vi "Merge 2 lines in array.vi"(8 "Index of 2nd line to merge":i32, 9 "Index of 1st line to merge":i32, 11 "Lines":T1[](array[typedef])) -> (3 "Merged Lines":T1[](array[typedef]))   [LabVIEW 2017]
uses:
  Vector Library/Line.ctl
  Vector Library/Vector.ctl
panel:
  out "Line to Merge":cluster{"Points":cluster{"X":dbl, "Y":dbl}[]}
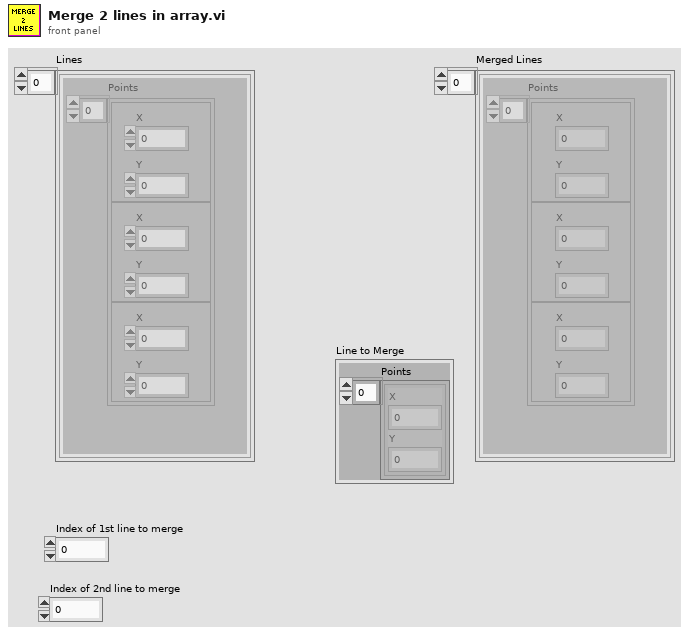
[diagram p1: front panel]
types:
  T1 = typedef "Line.ctl" = cluster{"Points":T2[]}
  T2 = typedef "Vector.ctl" = cluster{"X":dbl, "Y":dbl}
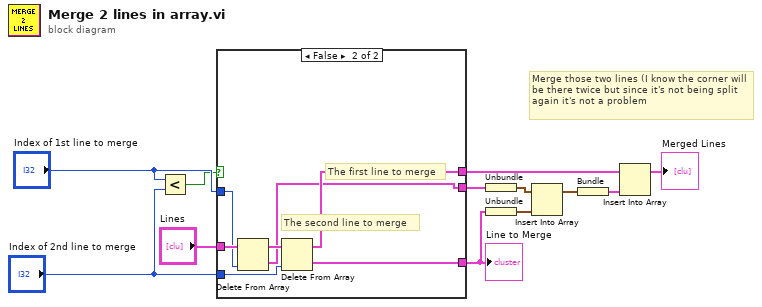
[diagram p0: block diagram]
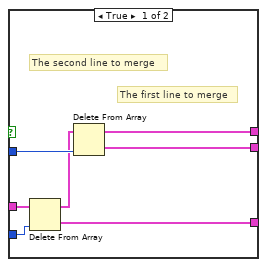
[diagram p2: hidden frame]
diagram:
  # "Merge those two lines (I know the corner will be there twice but since it's not being split again it's not a problem"
  n1 = Less?(x="Index of 1st line to merge", y="Index of 2nd line to merge") -> (x < y?=w4:bool)
  n2 = case shown="False" w4 {
    tunnel: "Lines" -> [w19 w23]
    tunnel: [w14 w20] -> w11
    tunnel: [w18 w26] -> w9
    tunnel: [w13 w25] -> w3
    tunnel: "Index of 1st line to merge" -> [w16 w22]
    tunnel: "Index of 2nd line to merge" -> [w17 w24]
    frame True {
      # "The first line to merge"
      # "The second line to merge"
      n3 = Delete From Array(array=w19, index=w17) -> (deleted portion=w18:T1, array with subset deleted=w15:T1[])  [unwired: 1 in]
      n4 = Delete From Array(array=w15, index=w16) -> (deleted portion=w14:T1, array with subset deleted=w13:T1[])  [unwired: 1 in]
    }
    frame False {
      # "The first line to merge"
      # "The second line to merge"
      n5 = Delete From Array(array=w23, index=w22) -> (deleted portion=w20:T1, array with subset deleted=w21:T1[])  [unwired: 1 in]
      n6 = Delete From Array(array=w21, index=w24) -> (deleted portion=w26:T1, array with subset deleted=w25:T1[])  [unwired: 1 in]
    }
  }
  "Line to Merge" <- w9
  n7 = Unbundle(w11) -> ("Points"=w10:T2[])
  n8 = Unbundle(w9) -> ("Points"=w8:T2[])
  n9 = Insert Into Array(array=w10, new element=w8) -> (w7:T2[])  [unwired: 1 in]
  n10 = Bundle("Points"=w7) -> (w2:cluster{"Points":T2[]})  [unwired: 1 in]
  n11 = Insert Into Array(array=w3, new element=w2) -> (→"Merged Lines":T1[])  [unwired: 1 in]
